vi "BuildConstructor.vi"(7 "PythonConverter_BD in":refnum<class "PyConvBD.lvclass">, 8 "error in":errorcluster, 11 "Function in":refnum<class "NamedUnbundler.lvclass">) -> (0 "error out":errorcluster, 3 "Function out":refnum<class "NamedUnbundler.lvclass">, 4 "constructor":string, 5 "PythonConverter_BD out":refnum<class "PyConvBD.lvclass">)   [LabVIEW 2014, in "NamedUnbundler.lvclass"]
uses:
  NamedUnbundler.lvclass
  Python/PythonConverter_BD/PyConvBD.lvclass
  Python/Parsing/Classes/PythonFunction/PythonFunction.lvclass/PythonFunction.ctl
  Python/Parsing/Classes/PythonFunction/PythonFunction.lvclass
  GrowableFunction/GrowableFunction.lvclass
  Python/Parsing/Python Functions.lvlib
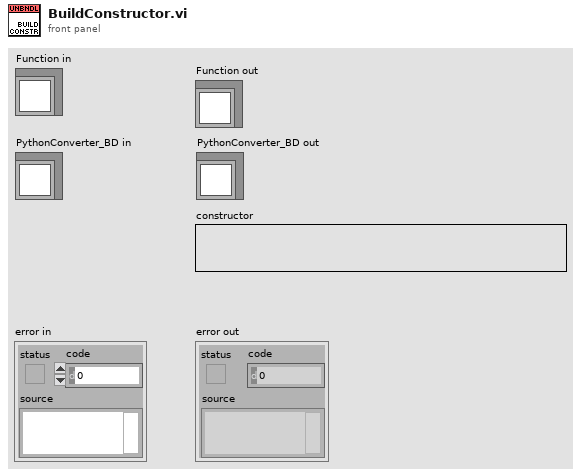
[diagram p1: front panel]
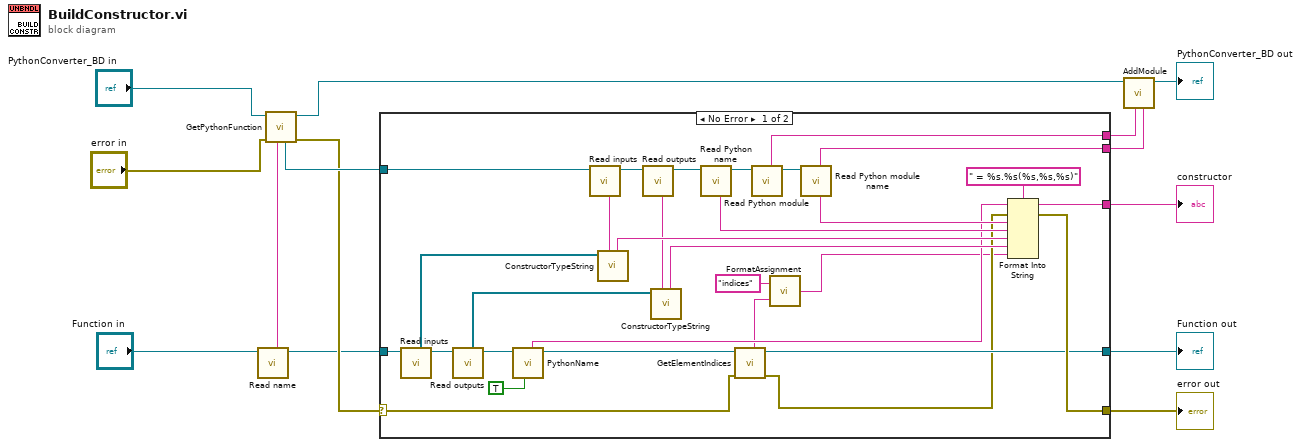
[diagram p0: block diagram]
diagram:
  n1 = call-dynamic "Read name.vi"("Node in"="Function in") -> ("Node out"=w8:refnum<class "NamedUnbundler.lvclass">, "name"=w9:string)  [unwired: 7 in]
  n2 = call "GetPythonFunction.vi"("function name"=w9, "error in"="error in", "PythonConverter_BD in"="PythonConverter_BD in") -> ("error out"=w13:errorcluster, "PythonConverter_BD out"=w12:refnum<class "PyConvBD.lvclass">, "Python function"=w14:refnum<class "PythonFunction.lvclass">)  [unwired: 4 in]
  n3 = case shown="No Error" w13 {
    selector: w13 -> [w19 w45]
    tunnel: [w39 w45] -> w4
    tunnel: [w38 _] -> w1
    tunnel: w14 -> [w29 _]
    tunnel: [w37 _] -> w11
    tunnel: [w36 _] -> w10
    tunnel: w8 -> [w28 w44]
    tunnel: [w20 w44] -> w6
    frame No Error {
      n4 = call-dynamic "Read inputs.vi"("Node in"=w28) -> ("Node out"=w26:refnum<class "NamedUnbundler.lvclass">, "inputs"=w27:refnum<class "Terminal.lvclass">[])  [unwired: 7 in]
      n5 = call-dynamic "Read outputs.vi"("Node in"=w26) -> ("Node out"=w24:refnum<class "NamedUnbundler.lvclass">, "outputs"=w25:refnum<class "Terminal.lvclass">[])  [unwired: 7 in]
      n6 = call-dynamic "PythonName.vi"("add self"=TRUE, "Node in"=w24) -> ("Node out"=w21:refnum<class "NamedUnbundler.lvclass">, "name"=w23:string)  [unwired: 6 in, 2 out]
      n7 = call "Read inputs.vi"("PythonFunction in"=w29) -> ("PythonFunction out"=w30:refnum<class "PythonFunction.lvclass">, "inputs"=w31:string)  [unwired: 7 in]
      n8 = call "ConstructorTypeString.vi"("list"=w31, "terminals"=w27) -> ("constructor string"=w42:string)  [unwired: 7 in]
      n9 = call "Read outputs.vi"("PythonFunction in"=w30) -> ("PythonFunction out"=w32:refnum<class "PythonFunction.lvclass">, "outputs"=w33:string)  [unwired: 7 in]
      n10 = call "ConstructorTypeString.vi"("list"=w33, "terminals"=w25) -> ("constructor string"=w41:string)  [unwired: 7 in]
      n11 = call "Read Python name.vi"("PythonFunction in"=w32) -> ("PythonFunction out"=w35:refnum<class "PythonFunction.lvclass">, "Python name"=w43:string)  [unwired: 7 in]
      n12 = call "GetElementIndices.vi"("error in"=w19, "NamedBundler in"=w21) -> ("error out"=w18:errorcluster, "NamedBundler out"=w20:refnum<class "NamedUnbundler.lvclass">, "indices"=w17:string)  [unwired: 5 in]
      n13 = call "Read Python module.vi"("PythonFunction in"=w35) -> ("PythonFunction out"=w34:refnum<class "PythonFunction.lvclass">, "Python module"=w37:string)  [unwired: 7 in]
      n14 = call "FormatAssignment.vi"("value"=w17, "name"="indices") -> ("python assignment"=w16:string)
      n15 = call "Read Python module  name.vi"("PythonFunction in"=w34) -> ("Python module  name"=w36:string)  [unwired: 7 in, 1 out]
      n16 = Format Into String(format string=" = %s.%s(%s,%s,%s)", initial string=w23, error in=w18, w36, w43, w42, w41, w16) -> (resulting string=w38:string, error out=w39:errorcluster)
    }
    frame Error {
    }
  }
  "error out" <- w4
  "Function out" <- w6
  "constructor" <- w1
  n17 = call "AddModule.vi"("python module name"=w10, "python module"=w11, "PythonConverter_BD in"=w12) -> ("PythonConverter_BD out"=→"PythonConverter_BD out":refnum<class "PyConvBD.lvclass">)  [unwired: 5 in, 1 out]
